vi "multiFeature.vi"(11 "Shared_strings":string[][](array[string])) -> ()   [LabVIEW 2018]
uses:
  Global Variables.vi
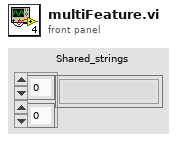
[diagram p1: front panel]
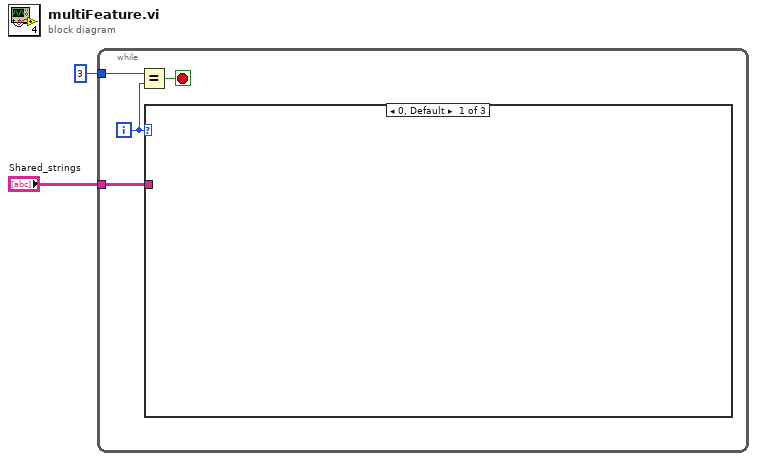
[diagram p0: block diagram]
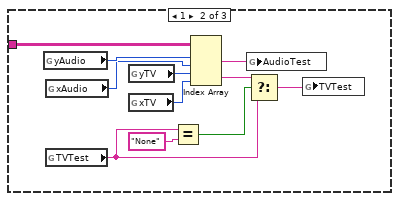
[diagram p2: hidden frame]
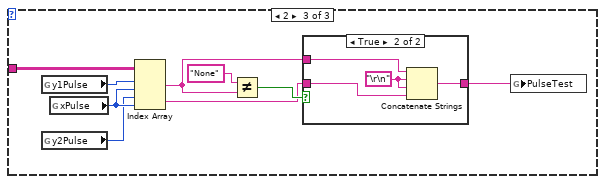
[diagram p3: hidden frame]
diagram:
  n1 = while {
    tunnel: "Shared_strings" -> [w4]
    tunnel: 3 -> [w3]
    i -> [w5]
    stop <- w6 stop-if-true
    n2 = Equal?(x=w3, y=w5) -> (x = y?=w6:bool)
    n3 = case shown="0, Default" w5 {
      tunnel: w4 -> [_ w17 w25]
      frame 0, Default {
      }
      frame 1 {
        n4 = global read "Global Variables.vi" "yAudio"() -> (w16:i32)
        n5 = global read "Global Variables.vi" "xAudio"() -> (w15:i32)
        n6 = global read "Global Variables.vi" "TVTest"() -> (w10:string)
        n7 = global read "Global Variables.vi" "yTV"() -> (w14:i32)
        n8 = global read "Global Variables.vi" "xTV"() -> (w13:i32)
        n9 = Equal?(x=w10, y="None") -> (x = y?=w9:bool)
        n10 = Index Array(array=w17, index (row) #1=w16, index (col) #1=w15, index (row) #2=w14, index (col) #2=w13) -> (element #1=w12:string, element #2=w11:string)
        n11 = global write "Global Variables.vi" "AudioTest"(w12) -> ()
        n12 = Select(t=w11, s=w9, f=w10) -> (s? t:f=w8:string)
        n13 = global write "Global Variables.vi" "TVTest"(w8) -> ()
      }
      frame 2 {
        n14 = global read "Global Variables.vi" "y1Pulse"() -> (w26:i32)
        n15 = global read "Global Variables.vi" "y2Pulse"() -> (w23:i32)
        n16 = global read "Global Variables.vi" "xPulse"() -> (w24:i32)
        n17 = Index Array(array=w25, index (row) #1=w26, index (col) #1=w24, index (row) #2=w23, index (col) #2=w24) -> (element #1=w18:string, element #2=w19:string)
        n18 = Not Equal?(x="None" ("search string"), y=w18) -> (x != y?=w21:bool)
        n19 = case shown="True" w21 {
          tunnel: [w27 w30] -> w20
          tunnel: w19 -> [w27 w28]
          tunnel: w18 -> [_ w29]
          frame False {
          }
          frame True {
            w31 = "\r\n"
            n20 = Concatenate Strings(w29, w31, w31, w28) -> (w30:string)
          }
        }
        n21 = global write "Global Variables.vi" "PulseTest"(w20) -> ()
      }
    }
  }
